vi "Encoder Read.vi"(8 "error in (no error)":errorcluster, 11 "Encoder Info":T1) -> (0 "error out":errorcluster, 2 "Rate":dbl, 3 "Distance":dbl, 4 "Stopped":bool, 5 "Direction":bool)   [LabVIEW 2014]
uses:
  Encoder Info.ctl
  <vilib>/Rock Robotics/WPI/Encoder/WPI_EncoderDevRef.ctl
  <vilib>/Rock Robotics/SystemInterfaces/Encoder/FPGA_EncoderIdx.ctl
  <vilib>/Rock Robotics/SystemInterfaces/Counter/FPGA_CounterCtrSystemIndex.ctl
  <vilib>/Rock Robotics/WPI/Encoder/WPI_EncoderType.ctl
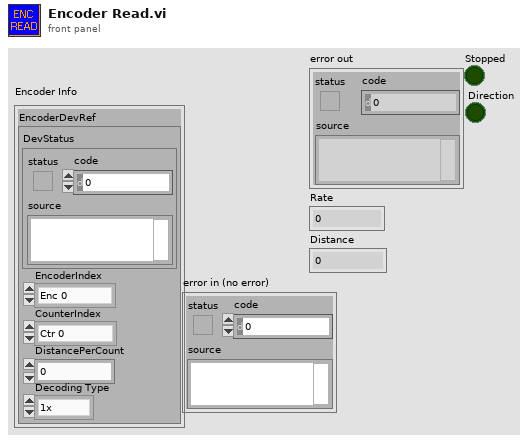
[diagram p1: front panel]
types:
  T1 = typedef "Encoder Info.ctl" = cluster{"EncoderDevRef":T2}
  T2 = typedef "WPI_EncoderDevRef.ctl" = cluster{"DevStatus":errorcluster, "EncoderIndex":T3, "CounterIndex":T4, "DistancePerCount":dbl, "Decoding Type":T5}
  T3 = typedef "FPGA_EncoderIdx.ctl" = enum8{"Enc 0", "Enc 1", "Enc 2", "Enc 3", "Enc 4", "Enc 5", "Enc 6", "Enc 7", "Invalid"}
  T4 = typedef "FPGA_CounterCtrSystemIndex.ctl" = enum8{"Ctr 0", "Ctr 1", "Ctr 2", "Ctr 3", "Ctr 4", "Ctr 5", "Ctr 6", "Ctr 7", "Invalid"}
  T5 = typedef "WPI_EncoderType.ctl" = enum16{"1x", "2x", "4x"}
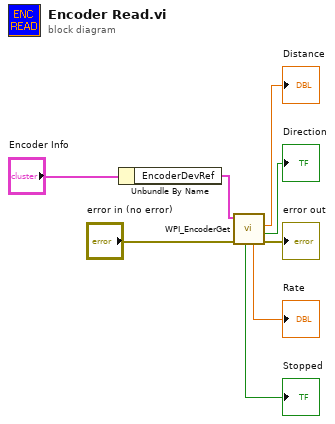
[diagram p0: block diagram]
diagram:
  n1 = Unbundle By Name("Encoder Info") -> ("EncoderDevRef"=w7:T2)
  n2 = call <vilib>:"WPI_EncoderGet.vi"("error in (no error)"="error in (no error)", "EncoderDevRef"=w7) -> ("error out"=→"error out":errorcluster, "Direction"=→"Direction":bool, "Distance"=→"Distance":dbl, "Rate"=→"Rate":dbl, "Stopped"=→"Stopped":bool)  [unwired: 4 in, 1 out]
